vi "Unregister HTTP Handler.vi"(8 "error in (no error)":errorcluster, 10 "Handler":refnum<class "Handler.lvclass">, 11 "VolatusAPI in":refnum<class "VolatusAPI.lvclass">) -> (0 "error out":errorcluster, 3 "VolatusAPI out":refnum<class "VolatusAPI.lvclass">)   [LabVIEW 2020, in "Volatus.lvlib" / "VolatusAPI.lvclass"]
uses:
  VolatusAPI.lvclass
  VolatusAPI.lvclass/VolatusAPI.ctl
  lv-vecto/Vecto/Vecto/Vecto.lvclass
  lv-http-server/HTTP Server/Server/Server.lvclass
  lv-http-server/HTTP Server/Handler/Handler.lvclass
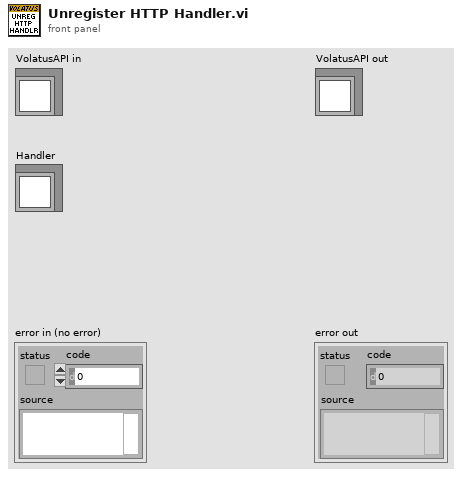
[diagram p1: front panel]
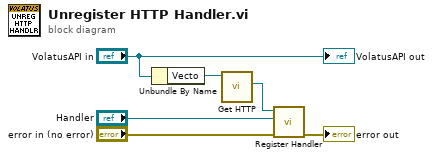
[diagram p0: block diagram]
diagram:
  n1 = Unbundle By Name("VolatusAPI in") -> ("Vecto"=w5:refnum<class "Vecto.lvclass">)
  n2 = call "Get HTTP.vi"("Vecto in"=w5) -> ("HTTP"=w4:refnum<class "Server.lvclass">)  [unwired: 8 in, 2 out]
  n3 = call "Register Handler.vi"("error in (no error)"="error in (no error)", "Handler"="Handler", "Server in"=w4) -> ("error out"=→"error out":errorcluster)  [unwired: 7 in, 1 out]
  "VolatusAPI out" <- "VolatusAPI in"
